vi "Copy Scripting .LLB to LV Addons dir.vi"(5 "Files Generated by Build":path[](array[path]), 6 "Top Level/Always Included VIs":path[](array[path]), 7 "Destination Path":path, 8 "error in (no error)":errorcluster, 9 "Target Name":string, 10 "Build Specification Name":string, 11 "Project Path":path) -> (0 "error out":errorcluster)   [LabVIEW 2019]
doc: "This VI is called after each run of a build specification. The VI will copy the generated LLB (Engine or System Explorer) into the VeriStand Custom Device folder (...\\Documents\\National Instruments\\NI VeriStand 2013...)."
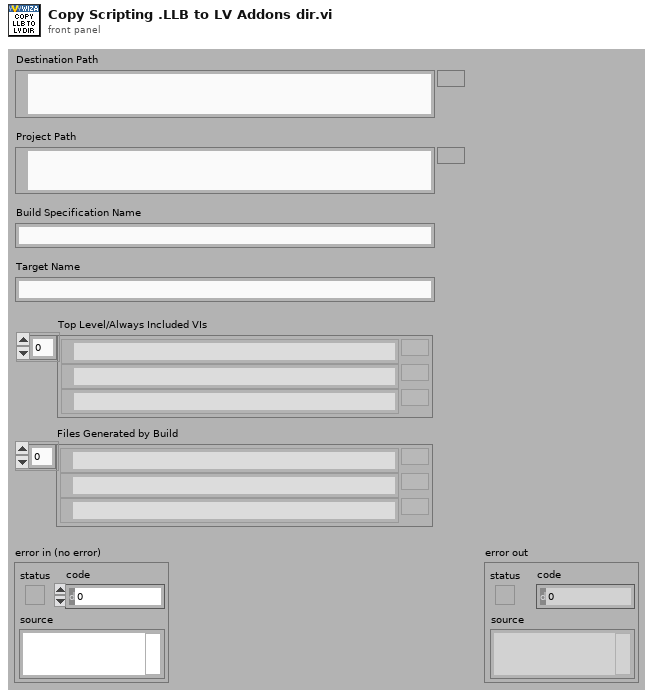
[diagram p1: front panel]
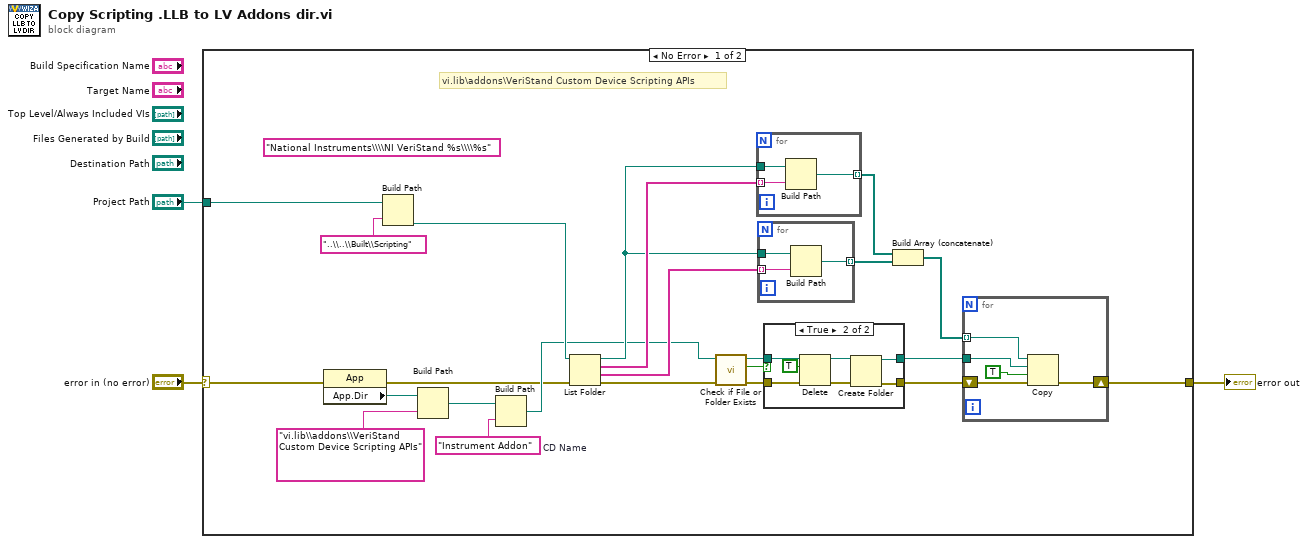
[diagram p0: block diagram]
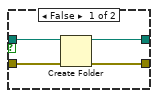
[diagram p2: hidden frame]
diagram:
  n1 = case shown="No Error" "error in (no error)" {
    selector: "error in (no error)" -> [w15 w49]
    tunnel: [w16 w49] -> w1
    tunnel: "Project Path" -> [w13 _]
    frame No Error {
      w4 = "Instrument Addon"  # CD Name
      (unwired) "National Instruments\\\\NI VeriStand %s\\\\%s" ("name or relative path")
      # "vi.lib\\addons\\VeriStand Custom Device Scripting APIs"
      n2 = property class="App"(error in=w15) -> (error out=w5:errorcluster, "App.Dir"=w9:path)  [unwired: 1 in, 1 out]
      n3 = Build Path(base path=w13, name or relative path="..\\..\\Built\\Scripting") -> (appended path=w10:path)
      n4 = Build Path(base path=w9, name or relative path="vi.lib\\addons\\VeriStand Custom Device Scripting APIs") -> (appended path=w7:path)
      n5 = Build Path(base path=w7, name or relative path=w4) -> (appended path=w6:path)
      n6 = List Folder(path=w10, error in=w5) -> (path out=w19:path, filenames=w26:string[], folder names=w20:string[], error out=w17:errorcluster)  [unwired: 2 in]
      n7 = call <vilib>:"Check if File or Folder Exists.vi"("error in (no error)"=w17, "path"=w6) -> ("error out"=w21:errorcluster, "file or folder exists?"=w23:bool, "dup path"=w22:path)  [unwired: 7 in]
      n8 = for {
        tunnel: w26 -> [w47] mode=indexing
        tunnel: w19 -> [w48]
        tunnel: [w46] -> w25 mode=indexing
        n9 = Build Path(base path=w48, name or relative path=w47) -> (appended path=w46:path)
      }
      n10 = for {
        tunnel: w20 -> [w44] mode=indexing
        tunnel: w19 -> [w45]
        tunnel: [w43] -> w18 mode=indexing
        n11 = Build Path(base path=w45, name or relative path=w44) -> (appended path=w43:path)
      }
      n12 = case shown="True" w23 {
        tunnel: w22 -> [w30 w37]
        tunnel: w21 -> [w29 w36]
        tunnel: [w28 w32] -> w12
        tunnel: [w27 w31] -> w11
        frame False {
          n13 = Create Folder(path (use dialog)=w30, error in=w29) -> (created path=w28:path, error out=w27:errorcluster)  [unwired: 1 in, 1 out]
        }
        frame True {
          n14 = Delete(path (use dialog)=w37, entire hierarchy (F)=TRUE, error in=w36) -> (deleted path=w35:path, error out=w34:errorcluster)  [unwired: 2 in, 1 out]
          n15 = Create Folder(path (use dialog)=w35, error in=w34) -> (created path=w32:path, error out=w31:errorcluster)  [unwired: 1 in, 1 out]
        }
      }
      n16 = Build Array (concatenate)(w25, w18) -> (w24:path[])
      n17 = for {
        tunnel: w24 -> [w39] mode=indexing
        shift-right: [w40] -> w16
        shift-left: w11 -> [w41]
        tunnel: w12 -> [w38]
        n18 = Copy(8:w41, 9:TRUE ("overwrite (F)"), 10:w38, 11:w39) -> (0:w40:errorcluster)  [unwired: 1 in, 2 out]
      }
    }
    frame Error {
    }
  }
  "error out" <- w1
